vi "GlobalLogger.vi"(8 "error in (no error)":errorcluster, 10 "Enum":enum16{"Get", "Set"}(ring), 11 "Logger in":refnum<class "Logger.lvclass">) -> (0 "error out":errorcluster, 3 "Logger":refnum<class "Logger.lvclass">)   [LabVIEW 2014]
uses:
  Logger/Logger.lvclass
  OperationErrorType.ctl
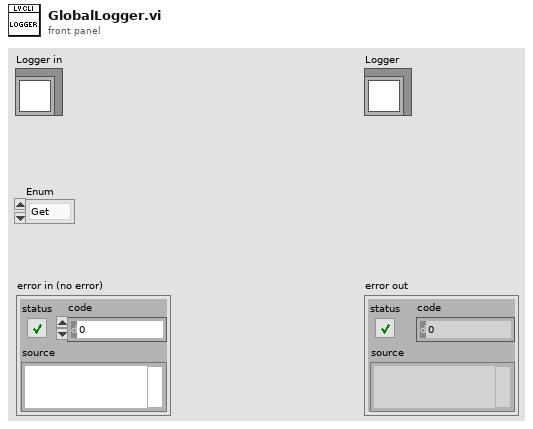
[diagram p1: front panel]
types:
  T1 = typedef "OperationErrorType.ctl" = enum16{"RequiredArgumentMissing", "UnknownArguments", "LoggerSetMultipleTimes", "OperationBrokenError"}
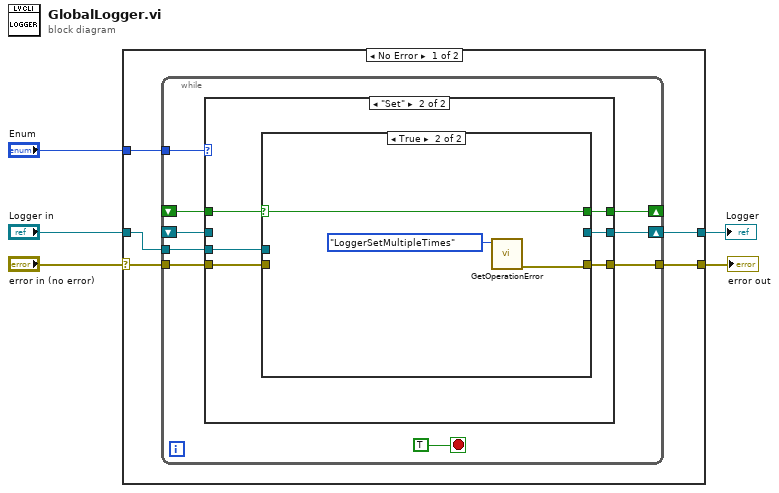
[diagram p0: block diagram]
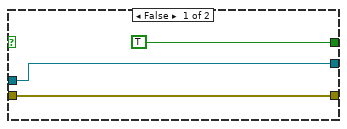
[diagram p3: hidden frame]
diagram:
  n1 = case shown="No Error" "error in (no error)" {
    selector: "error in (no error)" -> [w7 w35]
    tunnel: "Enum" -> [w10 _]
    tunnel: "Logger in" -> [w9 w36]
    tunnel: [w8 w36] -> w4
    tunnel: [w6 w35] -> w2
    frame No Error {
      n2 = while {
        tunnel: w10 -> [w18]
        tunnel: w9 -> [w17]
        shift-right: [w16] -> w8
        shift-left: _ -> [w15]
        tunnel: w7 -> [w13]
        shift-right: [w11] -> _
        shift-left: _ -> [w14]
        tunnel: [w12] -> w6
        stop <- TRUE stop-if-true
        n3 = case shown="\"Set\"" w18 {
          tunnel: w17 -> [_ w23]
          tunnel: [w22 w24] -> w16
          tunnel: w15 -> [w22 _]
          tunnel: w14 -> [w20 w25]
          tunnel: w13 -> [w21 w28]
          tunnel: [w21 w27] -> w12
          tunnel: [w20 w26] -> w11
          frame "Get" {
          }
          frame "Set" {
            n4 = case shown="True" w25 {
              selector: w25 -> [_ w34]
              tunnel: w28 -> [w31 _]
              tunnel: [w31 w33] -> w27
              tunnel: [TRUE w34] -> w26
              tunnel: [w29 _] -> w24
              tunnel: w23 -> [w29 _]
              frame False {
              }
              frame True {
                n5 = call "GetOperationError.vi"("Operation Error Type"=OperationErrorType."LoggerSetMultipleTimes") -> ("error out"=w33:errorcluster)  [unwired: 10 in]
              }
            }
          }
        }
      }
    }
    frame Error {
    }
  }
  "Logger" <- w4
  "error out" <- w2
